vi "InsertEphys.vi"(8 "error in (no error)":errorcluster, 9 "ephys_path":path, 10 "ephys_start_time":timestamp, 11 "connection reference":T1) -> (0 "error out":errorcluster, 3 "EphysPK":T2)   [LabVIEW 2014]
uses:
  <vilib>/addons/database/NI_Database_API.lvlib
  EphysPrimary.ctl
  SessionPrimary.ctl
  <vilib>/addons/database/Connection.llb/Conn ObjectReference.ctl
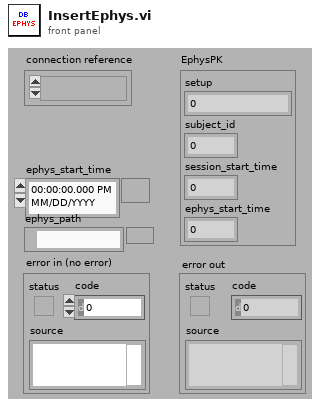
[diagram p1: front panel]
types:
  T1 = typedef "NI_Database_API.lvlib/Conn ObjectReference.ctl" = refnum<k1>
  T2 = typedef "EphysPrimary.ctl" = cluster{"setup":u8, "subject_id":i32, "session_start_time":dbl, "ephys_start_time":dbl}
  T3 = cluster{"setup":u8, "session_start_time":timestamp, "ephys_start_time":timestamp, "ephys_path":path}
  T4 = typedef "SessionPrimary.ctl" = cluster{"setup":u8, "subject_id":i32, "session_start_time":dbl}
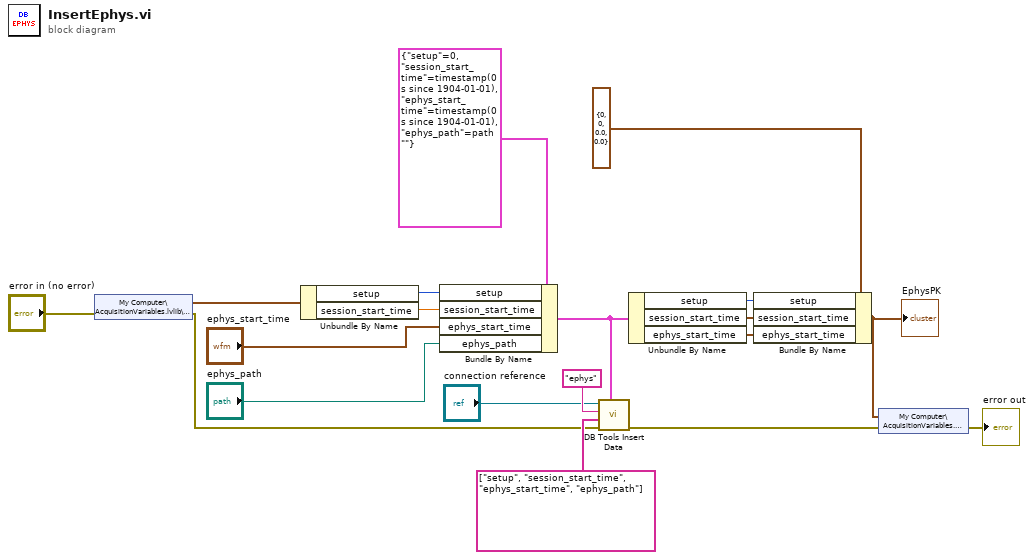
[diagram p0: block diagram]
diagram:
  n1 = shared-variable "My Computer\\AcquisitionVariables.lvlib\\SessionPK"(error in="error in (no error)") -> (w6:T4, error out=w5:errorcluster)
  n2 = Unbundle By Name(w6) -> ("setup"=w16:u8, "session_start_time"=w15:dbl)
  n3 = Bundle By Name(cluster=T3 {"setup"=0, "session_start_time"=timestamp(0 s since 1904-01-01), "ephys_start_time"=timestamp(0 s since 1904-01-01), "ephys_path"=path ""} ("Cluster"), "setup"=w16, "session_start_time"=w15, "ephys_start_time"="ephys_start_time", "ephys_path"="ephys_path") -> (w11:T3)
  n4 = call <vilib>:"DB Tools Insert Data.vi"("data"=w11, "error in (no error)"=w5, "columns"=string[] ["setup", "session_start_time", "ephys_start_time", "ephys_path"], "table"="ephys", "connection reference"="connection reference") -> ("error out"=w1:errorcluster)  [unwired: 5 in, 1 out]
  n5 = Unbundle By Name(w11) -> ("setup"=w10:u8, "session_start_time"=w9:timestamp, "ephys_start_time"=w8:timestamp)
  n6 = Bundle By Name(cluster=T2 {"setup"=0, "subject_id"=0, "session_start_time"=0.0, "ephys_start_time"=0.0} ("EphysPK"), "setup"=w10, "session_start_time"=w9, "ephys_start_time"=w8) -> (w3:T2)
  "EphysPK" <- w3
  n7 = shared-variable "My Computer\\AcquisitionVariables.lvlib\\EphysPK"(w3, error in=w1) -> (error out=→"error out":errorcluster)
